vi "Laurel GET Data.vi"(6 "byte count":i32=9, 7 "Use Delay":bool, 8 "error in (no error)":errorcluster, 11 "Laurel IP Address":string) -> (0 "error out":errorcluster, 2 "Gallons (Item 2)":dbl, 3 "Flow Rate (Item 1)":dbl)   [LabVIEW 2016]
uses:
  Type Definitions/Laurel Serial Commands.ctl
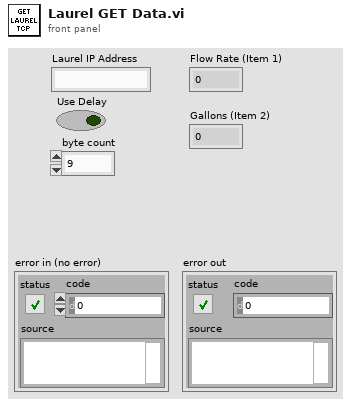
[diagram p1: front panel]
types:
  T1 = typedef "Laurel Serial Commands.ctl" = string
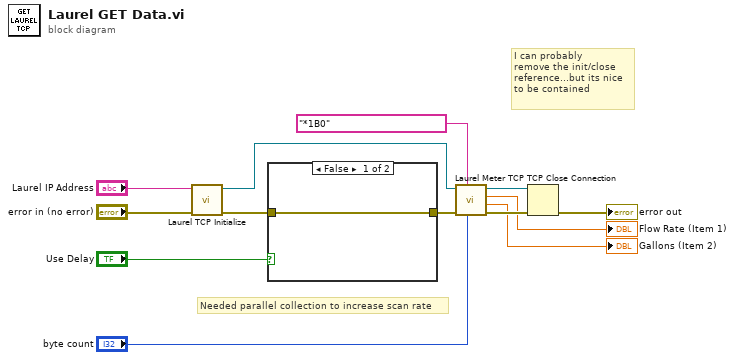
[diagram p0: block diagram]
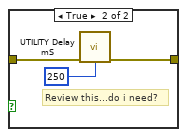
[diagram p2: hidden frame]
diagram:
  # "I can probably \nremove the init/close \nreference...but its nice \nto be contained"
  # "Needed parallel collection to increase scan rate"
  n1 = call "Laurel TCP Initialize.vi"("Error In"="error in (no error)", "Laurel IP Address"="Laurel IP Address") -> ("Error Out"=w10:errorcluster, "Laurel Ref"=w9:refnum<k5>)  [unwired: 8 in]
  n2 = case shown="False" "Use Delay" {
    tunnel: w10 -> [w14 w17]
    tunnel: [w14 w15] -> w4
    frame False {
    }
    frame True {
      # "Review this...do i need?"
      n3 = call "UTILITY Delay mS.vi"("Error In"=w17, "milliseconds to wait"=u32 250) -> ("Error Out"=w15:errorcluster)  [unwired: 13 in]
    }
  }
  n4 = call "Laurel Meter TCP.vi"("byte count (Individual)"="byte count", "Laurel Serial Commands"=T1 "*1B0", "error in (no error)"=w4, "TCP Network Connection in"=w9) -> ("error out"=w11:errorcluster, "Gallons (Item 2)"=→"Gallons (Item 2)":dbl, "Flow Rate (Item 1)"=→"Flow Rate (Item 1)":dbl, "TCP Network Connection out"=w13:refnum<k5>)  [unwired: 2 in, 2 out]
  n5 = TCP Close Connection(connection ID=w13, error in (no error)=w11) -> (error out=→"error out":errorcluster)  [unwired: 1 in, 1 out]
